vi "MTM2_acceptCommand_setCorrectionMode.vi"(8 "error in (no error)":errorcluster, 11 "command_setCorrectionMode_Ctl":T1) -> (0 "error out":errorcluster, 2 "function return":i32, 3 "command_setCorrectionMode_Ctl out":T1)   [LabVIEW 2018, in "SALLV_MTM2.lvlib"]
doc: "int MTM2_shm_acceptCommand_setCorrectionModeLV(MTM2_command_setCorrectionModeLV *command_setCorrectionMode_Ctl );"
uses:
  SALLV_MTM2.lvlib
  DataTypes/command_setCorrectionMode.ctl
  SALLV_MTM2.so
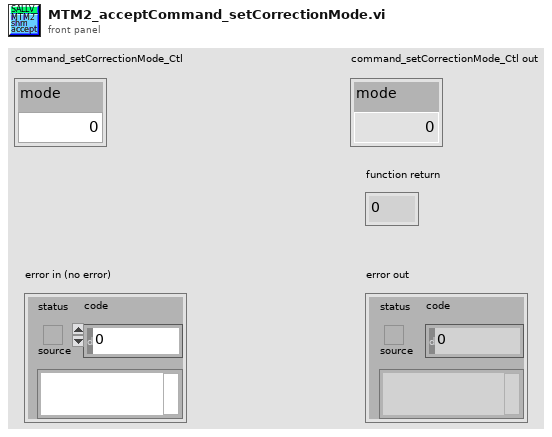
[diagram p1: front panel]
types:
  T1 = typedef "SALLV_MTM2.lvlib/command_setCorrectionMode.ctl" = cluster{"mode":i32}
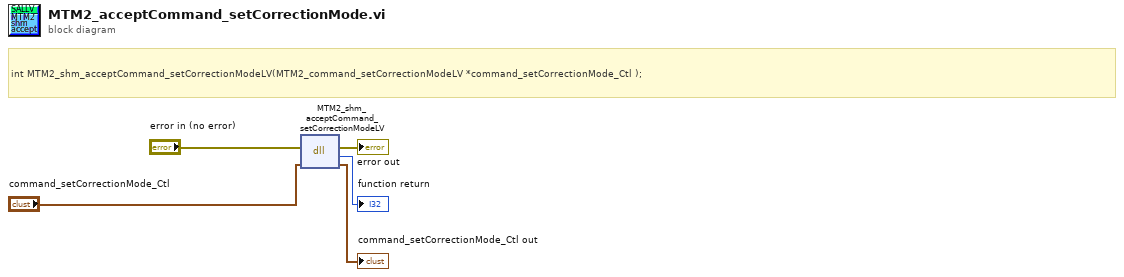
[diagram p0: block diagram]
diagram:
  # "int MTM2_shm_acceptCommand_setCorrectionModeLV(MTM2_command_setCorrectionModeLV *command_setCorrectionMode_Ctl );"
  n1 = dll-call lib="home/ttsai/Document/salApiMTM2/SALLV_MTM2/SALLV_MTM2.*" fn="MTM2_shm_acceptCommand_setCorrectionModeLV"(error in="error in (no error)", "command_setCorrectionMode_Ctl"="command_setCorrectionMode_Ctl") -> (error out=→"error out":errorcluster, →"function return":i32, "command_setCorrectionMode_Ctl"=→"command_setCorrectionMode_Ctl out":T1)  [unwired: 2 in, 1 out]
